vi "single sweep - adaptive - statistics.vi"(11 "x + iy":cdb[](array[numeric])) -> (0 "spot size":dbl, 1 "spot position":cdb, 2 "spot directed size":cdb)   [LabVIEW 2010]
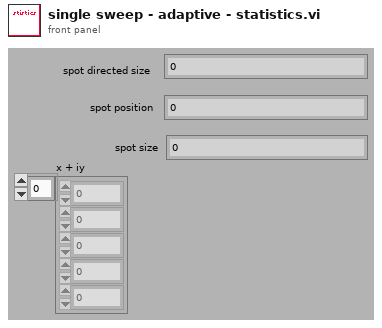
[diagram p1: front panel]
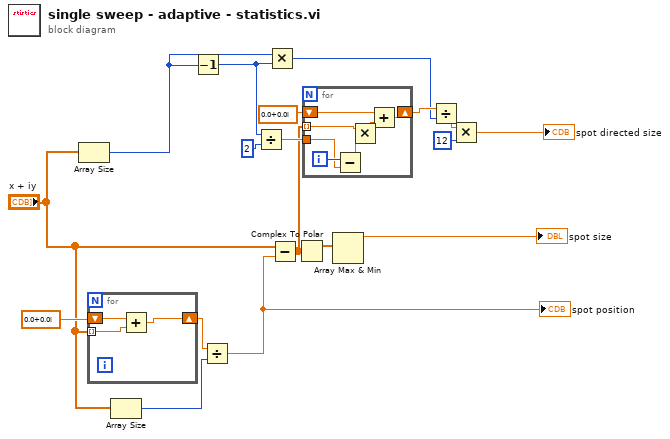
[diagram p0: block diagram]
diagram:
  n1 = Array Size(array="x + iy") -> (size(s)=w8:i32)
  n2 = for {
    shift-right: [w20] -> w5
    shift-left: cdb 0.0+0.0i -> [w21]
    tunnel: "x + iy" -> [w19] mode=indexing
    n3 = Add(x=w21, y=w19) -> (x+y=w20:cdb)
  }
  n4 = Array Size(array="x + iy") -> (size(s)=w4:i32)
  n5 = Decrement(x=w8) -> (x-1=w7:i32)
  n6 = Divide(x=w5, y=w4) -> (x/y=w1:cdb)
  "spot position" <- w1
  n7 = Divide(x=w7, y=2) -> (x/y=w17:dbl)
  n8 = Multiply(x=w8, y=w7) -> (x*y=w6:i32)
  n9 = Subtract(x="x + iy", y=w1) -> (x-y=w16:cdb[])
  n10 = Complex To Polar(r * e^(i*theta)=w16) -> (r=w18:dbl[])  [unwired: 1 out]
  n11 = for {
    tunnel: w17 -> [w27]
    tunnel: w16 -> [w26] mode=indexing
    shift-right: [w22] -> w13
    shift-left: cdb 0.0+0.0i -> [w23]
    i -> [w28]
    n12 = Subtract(x=w28, y=w27) -> (x-y=w25:dbl)
    n13 = Multiply(x=w26, y=w25) -> (x*y=w24:cdb)
    n14 = Add(x=w23, y=w24) -> (x+y=w22:cdb)
  }
  n15 = Array Max & Min(array=w18) -> (max value=→"spot size":dbl)  [unwired: 3 out]
  n16 = Divide(x=w13, y=w6) -> (x/y=w12:cdb)
  n17 = Multiply(x=w12, y=12) -> (x*y=→"spot directed size":cdb)
